vi "Test Report Contain Broken Error Type.vi"(8 "error in (no error)":errorcluster, 11 "XML Report Test in":refnum<class "XML Report Test.lvclass">) -> (0 "error out":errorcluster, 3 "XML Report Test out":refnum<class "XML Report Test.lvclass">)   [LabVIEW 2020, in "XML Report Test.lvclass"]
uses:
  XML Report Test.lvclass
  source/Plugins/XML Report/XML Report.lvclass
  source/Core/Result/Type.ctl
  source/Core/Result/Result.lvlib
  source/Core/Result/Status.ctl
  source/Core/Result/Result.ctl
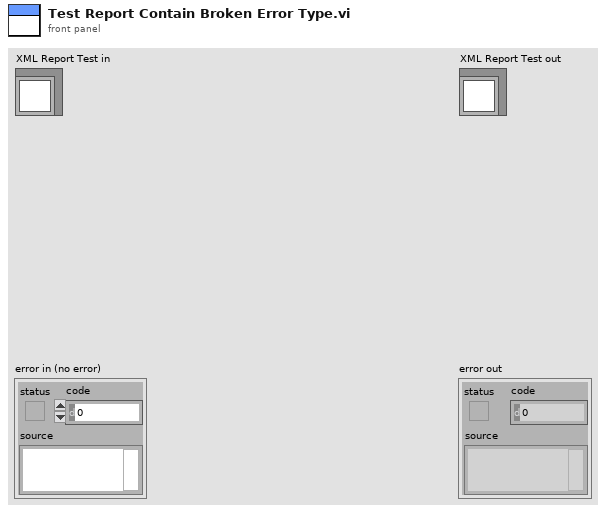
[diagram p1: front panel]
types:
  T1 = typedef "Result.lvlib/Result.ctl" = cluster{"Name":string, "Description":string, "Status":T2, "Result Type":T3, "Execution Time":dbl, "Data":cluster{"Expected":variant, "Actual":variant, "Delta":variant}}
  T2 = typedef "Result.lvlib/Status.ctl" = enum16{"", "Passed", "Failed", "Error", "Skipped", "Setup Error", "Broken", "Teardown Error"}
  T3 = typedef "Result.lvlib/Type.ctl" = enum16{"Test Case", "Test Suite", "Test Run", "Pass", "Fail", "Skip", "Pass if", "Fail if", "Pass if Error", "Fail if Error", "Pass if Equal", "Fail if Equal"}
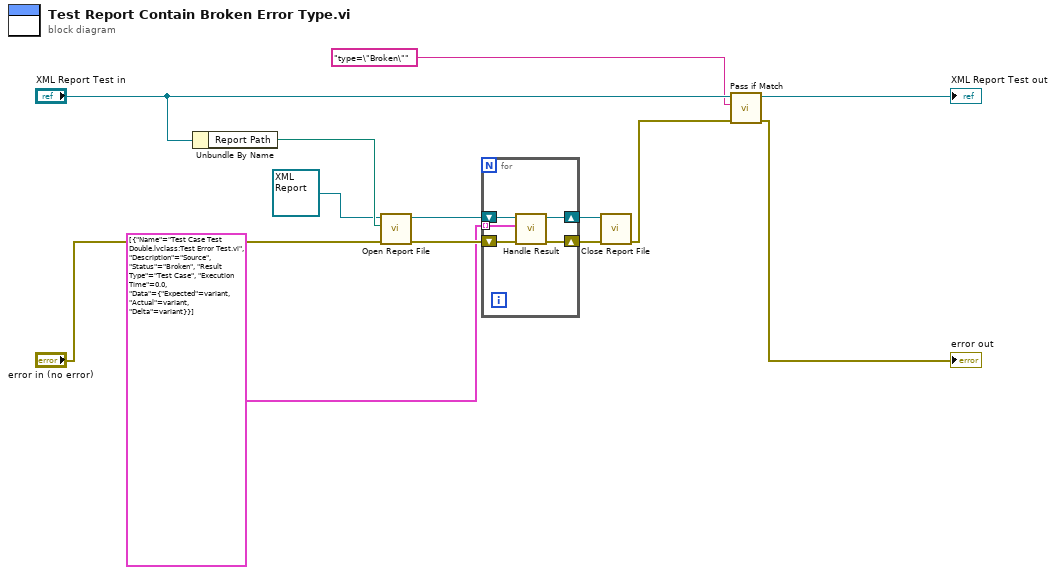
[diagram p0: block diagram]
diagram:
  n1 = Unbundle By Name("XML Report Test in") -> ("Report Path"=w7:path)
  n2 = call-dynamic "Open Report File.vi"("error in (no error)"="error in (no error)", "Report Path"=w7, "XML Report In"=refnum<class "XML Report.lvclass"> refnum) -> ("error out"=w13:errorcluster, "XML Report Out"=w3:refnum<class "XML Report.lvclass">)  [unwired: 7 in]
  n3 = for {
    tunnel: T1[] [{"Name"="Test Case Test Double.lvclass:Test Error Test.vi", "Description"="Source", "Status"=enum."Broken", "Result Type"=enum."Test Case", "Execution Time"=0.0, "Data"={"Expected"=variant, "Actual"=variant, "Delta"=variant}}] ("Data") -> [w14] mode=indexing
    shift-right: [w17] -> w4
    shift-left: w13 -> [w18]
    shift-right: [w15] -> w2
    shift-left: w3 -> [w16]
    n4 = call-dynamic "Handle Result.vi"("error in (no error)"=w18, "Result"=w14, "XML Report In"=w16) -> ("error out"=w17:errorcluster, "XML Report Out"=w15:refnum<class "XML Report.lvclass">)  [unwired: 7 in]
  }
  n5 = call-dynamic "Close Report File.vi"("error in (no error)"=w4, "XML Report In"=w2) -> ("error out"=w9:errorcluster)  [unwired: 8 in, 1 out]
  n6 = call "Pass if Match.vi"("error in (no error)"=w9, "regular expression"="type=\"Broken\"", "XML Report Test in"="XML Report Test in") -> ("error out"=→"error out":errorcluster, "XML Report Test out"=→"XML Report Test out":refnum<class "XML Report Test.lvclass">)  [unwired: 6 in, 1 out]
